vi "Comment Source.vi"(8 "Error In":errorcluster) -> (0 "Error Out":errorcluster)   [LabVIEW 2018, in "Tests.lvlib" / "Nodes.lvlib"]
uses:
  Nodes.lvlib
  src/Toolkit/Low-Level/Nodes/Comment/Comment.lvclass
  <vilib>/addons/_JKI Toolkits/Caraya/classes/Test/Test.lvclass
  <vilib>/addons/_JKI Toolkits/Caraya/classes/Assert/Assert.lvclass
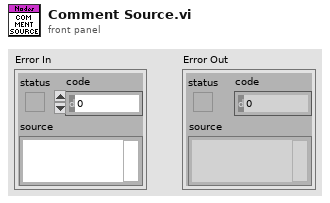
[diagram p1: front panel]
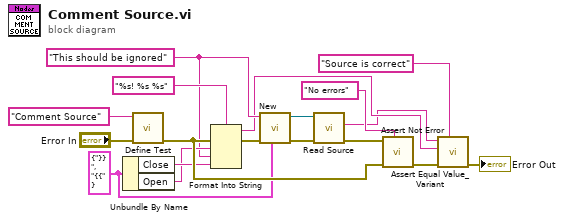
[diagram p0: block diagram]
diagram:
  w6 = cluster{"Close":string, "Open":string} {"Close"="}}", "Open"="{{"} ("Delimiters")
  w3 = "This should be ignored" ("Content")
  n1 = Unbundle By Name(w6) -> ("Close"=w5:string, "Open"=w4:string)
  n2 = call <vilib>:"Define Test.vi"("error in (no error)"="Error In", "Label (VI Title)"="Comment Source") -> ("error out"=w12:errorcluster)  [unwired: 9 in]
  n3 = Format Into String(format string="%s! %s %s", error in=w12, w4, w3, w5) -> (resulting string=w2:string, error out=w8:errorcluster)  [unwired: 1 in]
  n4 = call "New.vi"("Delimiters"=w6, "Error In"=w8, "Content"=w3) -> ("Error Out"=w10:errorcluster, "Comment"=w11:refnum<class "Comment.lvclass">)  [unwired: 7 in]
  n5 = call-dynamic "Read Source.vi"("Error In"=w10, "Node In"=w11) -> ("Error Out"=w9:errorcluster, "Source"=w1:string)  [unwired: 7 in, 1 out]
  n6 = call <vilib>:"Assert Not Error.vi"("Label"="No errors", "error in (no error)"=w12, "Not Error?"=w9) -> ("error out"=w15:errorcluster)  [unwired: 8 in]
  n7 = call <vilib>:"Assert Equal Value_Variant.vi"("Label"="Source is correct", "error in (no error)"=w15, "Y"=w2, "X"=w1) -> ("error out"=→"Error Out":errorcluster)  [unwired: 7 in]
